vi "Update I2C Messages Table.vi"(8 "error in (no error)":errorcluster, 10 "I2C Messages in":string[][](array[string]), 11 "I2C Table Ref":refnum<vi>) -> (0 "error out":errorcluster)   [LabVIEW 2025, in "I2C Bus Monitor UI.lvlib"]
uses:
  I2C Bus Monitor UI.lvlib
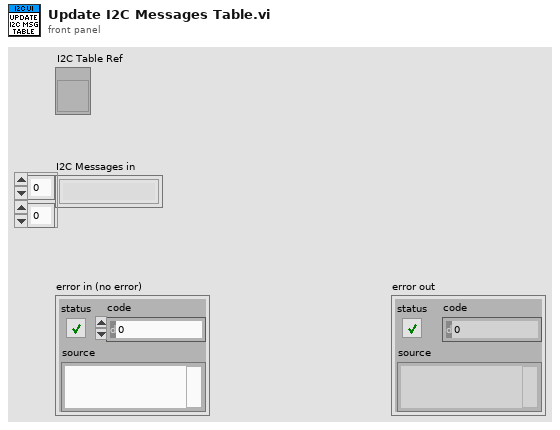
[diagram p1: front panel]
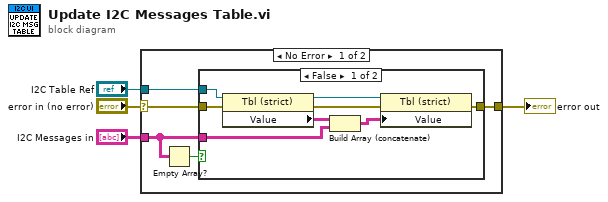
[diagram p0: block diagram]
diagram:
  n1 = case shown="No Error" "error in (no error)" {
    selector: "error in (no error)" -> [w8 w19]
    tunnel: "I2C Table Ref" -> [w9 _]
    tunnel: "I2C Messages in" -> [w5 _]
    tunnel: [w7 w19] -> w1
    frame No Error {
      n2 = Empty Array?(array=w5) -> (empty?=w6:bool)
      n3 = case shown="False" w6 {
        tunnel: w5 -> [w16 _]
        tunnel: w9 -> [w14 _]
        tunnel: w8 -> [w17 w18]
        tunnel: [w11 w18] -> w7
        frame False {
          n4 = property on="Property Node" class="Tbl (strict)"(reference=w14, error in=w17) -> (reference out=w12:refnum<vi>, error out=w10:errorcluster, "Value"=w13:string[][])
          n5 = Build Array (concatenate)(w13, w16) -> (w15:string[][])
          n6 = property on="Property Node" class="Tbl (strict)"(reference=w12, error in=w10, "Value"=w15) -> (error out=w11:errorcluster)  [unwired: 1 out]
        }
        frame True {
        }
      }
    }
    frame Error {
    }
  }
  "error out" <- w1
